vi "Query Input Attenuation.vi"(8 "error in (no error)":errorcluster, 9 "Attenuation Type (0:Current)":u16(ring) items=["Current", "MINimum", "MAXimum", "DEFault"], 10 "Platform Slot Number (10)":i16=10 min=-1 max=255, 11 "VISA resource name":refnum<visa-resource-name>) -> (0 "error out":errorcluster, 2 "Input Attenuation":dbl format="%#_6e", 3 "VISA resource name out":refnum<visa-resource-name>)   [LabVIEW 2018, in "LTB-1.lvlib" / "3150.lvlib"]
doc: "Queries the value indicating the current or the minimum/maximum absolute attenuation value, in dB."
uses:
  3150.lvlib
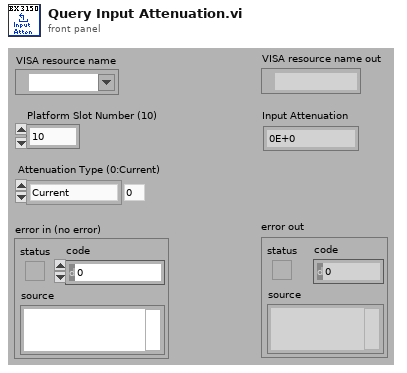
[diagram p1: front panel]
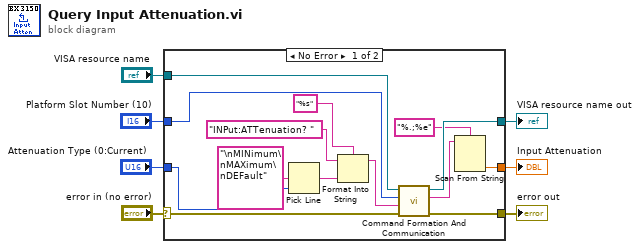
[diagram p0: block diagram]
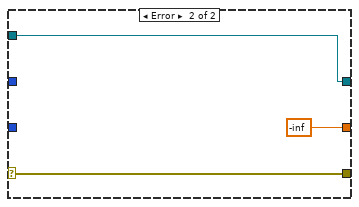
[diagram p2: hidden frame]
diagram:
  n1 = case shown="No Error" "error in (no error)" {
    selector: "error in (no error)" -> [w21 w24]
    tunnel: [w20 w24] -> w5
    tunnel: "VISA resource name" -> [w19 w23]
    tunnel: [w18 w23] -> w6
    tunnel: "Attenuation Type (0:Current)" -> [w15 _]
    tunnel: "Platform Slot Number (10)" -> [w12 _]
    tunnel: [w9 -inf] -> w1
    frame No Error {
      n2 = Pick Line(multi-line string="\nMINimum\nMAXimum\nDEFault" ("string (\"\")"), line index=w15) -> (output string=w14:string)  [unwired: 1 out]
      n3 = Format Into String(format string="%s", initial string="INPut:ATTenuation? " ("Command"), w14) -> (resulting string=w13:string)  [unwired: 1 in, 1 out]
      n4 = call "Command Formation And Communication.vi"("error in (no error)"=w21, "Command"=w13, "Platform Slot Number"=w12, "VISA resource name"=w19) -> ("error out"=w20:errorcluster, "Response"=w11:string, "VISA resource name out"=w18:refnum<visa-resource-name>)  [unwired: 1 in, 4 out]
      n5 = Scan From String(format string="%.;%e", input string=w11) -> (output 1=w9:dbl)  [unwired: 2 in, 4 out]
    }
    frame Error {
    }
  }
  "VISA resource name out" <- w6
  "error out" <- w5
  "Input Attenuation" <- w1
